vi "Main_21a.vi"() -> ()   [LabVIEW 2023]
uses:
  Cluster_Node.ctl
  ENUM Tile Marks.ctl
panel:
  out "Array":T1[][](array[typedef])
  out "Start Point":T2
  out "Answer":i32
  in  "Puzzle":string="...................................................................................................................................\n.....#..#..#.#..#..#..#................##.#.......#....................#......#.##...........#.....##...................#........#.\n.....#.#.............#.............#.....#.........#..................................#......#....#...##...#.#........#......###...\n.......#...#................#.......#....#.....#...#.......................#......#...#.##...#.....#.........#.......#.#...........\n.##.............#...................#...#......#........#.........................#...#........#....#....#.........#..........#....\n.....#..##....#..#...#......##......#.................................................#.#.....#......#......#.#.##.................\n..............#......#......#................#.................#.................#................#..#...#........##.............#.\n..........##..........##.......#.#.....#..........#...#.........#.....................#....#....................#..#.....##..#..##.\n.#.#..#..#.#....#....#.....#...#.#.................................................#......................#..##..#.........#...#...\n.....................#.........#.......###..#......................#...........####........##.......#.#.#......#.#....##.....#...#.\n.#.#...#....#.........##...#...........#..##.......#.......#.......#................#.....#...#...#.#.....#..............##......#.\n................#...#..#.........#.##............................................#......##.....##.......#...#........#..#..#.......\n..#..#..####...###.#..........#........#.......#.............#.....#....#............#..#........##......##.......#.....#....#.....\n.......#..........#.......................#.............##..........#..#..........#.....#.............##.........#..............#..\n..................#.............##...........................#.#......##.......................##.....#.#.....#................#...\n.......#...................##........#...............................#..............#..#..#.#..#..........#........#...........#...\n...#..........#..#...#.#.#............................#......................#.......#......##...#...............#...#..#..........\n...#.#..........#.#.....#........#.....#...#.......................#.....#..#...............#.....#.#......#....##...#....#..###...\n...#.##........#..##...#..........#..#..................................#..#.#.#.........#...........#....#.....#...#.#.........#..\n.....#.......#........#..............#.##.............#..#........#....#.....#.............#....#.#.#........##........#...#..#....\n....#......##....##........#..#....##.................#......................#.#.#................#....#..###..#...#...............\n....#....#.#........#.......#........#...................#.....#.........#....#............##.........#..............#...........#.\n............#..#.##..................#..........##.........................#..#....#................#................#..#....#.....\n.##.##........#..###.......#....#......................##..#......#.....#...#..#...............##.#.....##........#................\n.......#..#........#.........#...................#..#.....##...............#.#.#...#..........#............#.....##.........#......\n...###.......#...............#...................#..#...##.........#.............##..#..........................#..#...#.....#.....\n..#..............##.........#..#...............................#........#......#.#....#..........#................##.#...#.........\n...#......#..#....#.........#..#..........##............#....#.........#....#..#......#.........#..#...........#...................\n.#...###.....................#.............#.......#......###..#...........#.........................#..#.......#.#..#.....#.......\n.###........#......##...#...........................##......#.........#.........#........#........#.....##..........#....#.........\n.......#........#..#......#..............#..........##...#...#...........................#...........#...#..#......#...........#...\n.#....#........#......#..##..................#....................#.................................#......#.....#..#.......#......\n...#........#.....#..##...#.#.............#...#.#.#.....#......#........#...........#....#...............#..#.....#.......#........\n....#....#...#.#....#................#..#......#........#.#........#..#.#..#..#.....#..#..................##...................#...\n.......##........#...#..............###.#....#....#..#....##...#....##.#............#..#.#...#............#...................#.#..\n..#......#.........#..#.................#...#.......#....#...#..............##...#..........#.#...........................#....#...\n..#......#..#...........................#...........#....#.............#.#.........#...#.........................##............#...\n.....#................#.........#.#.........#...........#.#............#..................#....#.........................#..#..#...\n......#...#....##...................#.................#..#........#..#..#.....................#.............#.......#..#......#....\n.............##.................#.......#.........#..#....#...#.......#...................#.........#.......##.#...................\n......#....#.................#..#....#..##..#............#..............#.............#.....#..#..#................#..#...#......#.\n..................#.........#.....................#......#....##..##...##..........#......#......#..#.............#.....#....#.....\n.......#...#..#....#..........#.......#.#.#...##.....##.#....#.##..................##........#...##..................#.............\n.............#...#..................#......##.........#.......##......#...#....##.....#...#..#...................#...####..........\n.............................#.......#....#........#..........#...#.......#.#............#..###........#...........#.#.............\n..........#...................#..#...............#.#..................#.....#...#..............................................##..\n.........................................#...#.#....#.......#........#..#......#.........#...............#.........................\n......#...#.......................#.....#................#.........#..#......#....................####.#..#.....................##.\n.......#...................#.##....#......#..........#...............##...#...#...............#.......#.....#.................#....\n....#.#...##............#.......#..........#..................#..........#.........#........#.........##...#.......................\n...#......#.........#........#....#.....#.........#....##....#..................#.......#.#.........#.#..................##....#...\n.....#................#.#...........#.............#..#.......#..........#..#...#.#.....###......##.....#.#.#.#.................#...\n.....................#..##.##...#...............#..#....#....#....#..####...#..................................#.........##..#.....\n.......##...............#......#.....#..........#..#..#.#.............#.....#......#.#.......#..................#............#..##.\n...#............#...#.........##............#...#...#......#.......#.....#...##...##...#...#................................#......\n...#.#.............................................##..............##..................#...........#...#..........#...........##...\n...#.#....................#......#....#.....##..........#.........#......#.#.......##.#.#....#.#....#.....#....##..................\n.............#...#.#..#......#........#.#...##.#...............#....#.........................#....#.......#.....##...#.........#..\n..................##..#..###......................#.......#.##.....#....#..#.....#....#..............#.....#.#..#....#.............\n.............#......#.###..###........#.#.#......#.#....#..#.......#..#............#.........#.#..#...............#.............##.\n.............#...#.............#.#.#..##..####..#......#.##.#...........##...##.............#......#.............#..#............#.\n..........#........#......#.#........#..............#......#..#.#.....#.................#...#...............#.#..........##........\n..............#.............##.....#............................#..........#..........#..#.....................#..#..#.............\n..........#...#.#.......##....#.......#..##......#...#.....#............#................#....#.......................#............\n....................#.....#..........#.......#.#........#...##..............#.....#.......#..##...#..#####.#.#.........##....#.....\n.................................................................S.................................................................\n........#.........##....#........#...........................##........#..............#........#.....#.#..............#....#.......\n......#............#.............#............#.##...........#..#.....#....#.....#......#.#.#.......#.#.#...#......................\n............................#.........#........###........#...#....#.........#................#..#.............#....#..............\n............#......##..##.##...##.............#.........#............#.###.....#..................##..................#..#.........\n..............#......#................#...............#.....##..#..........#.....#..#..........#...........#.......................\n.........................#...........#..#......#.............#..#....#.......#..#.....#...#.............................#........#.\n...........##.....##.................#..........#.#.#..............#.....#.........#............#.................#................\n.........................#......#.....#...#.##...........#......#....#....#......#..#.#..#..###..##.##.....#...................#...\n.....#...........#.....#.......#..##......##.#.#.#..........#..#..............#...#.#.#.....#............#.#....#..............#.#.\n...#...........#.........#..#.#.#.........#........#..#........................#..........#.............#....##.#...............#..\n...............#.....................................#..............................##...###.................#..#..........#.....#.\n........#..........#..#......###............#........................#..........#............................................#.....\n...............................#....................#..................................##.............#............................\n.........#............#..#..........#........#..#...##....#....#..#......#.....#.#...#......................##..................#..\n......##.#..........##.#..................................#.........#......##..#...............#........#.....#............#.......\n.........#..................#...........#.#.......................#..........#.......##.......#.....#...##...#........#...#.#......\n...#...................#.....#...........##............#..#...#..................#.#..........#........................#...........\n..#.........#.........#.........##...#.....#...........#.....................#....#............#..#.......#.........#.....#........\n..........#....#..........#.........#..........#..###........#.#..........##.................#......#...#..............#...........\n..#....##..........................#..........#........#.#..##..#.....#.#....#..#.....................#............#.#...........#.\n.....................................#..#.#..#...........#...#.#.......#........#...#.........#...#..#...............#.............\n.........#.#....##.................#.#.....#....#..#..#................#...##.......#...........#.....#.................##.........\n..#.........................#......#..............#.............#.......#.............#........#................#...###.#........#.\n.#..#............#..............#..#...........#................#.........#....#................#..#.............#.....#...#.....#.\n.....#.......................#............#...............#..........###.....##...........#..#...#.##.........#.......#............\n.#..#..........#.............................#......#.......##..........#.........#....#...#.....#..........#....#.................\n.........#.......................#.##.....#.....#.#....#.......##.....#....#......#.......#.#.....................#.##..#..#....#..\n.#......#.....#.....#.....................##.........#....#...##..#..................##...#.#.#..#........#..#.........#.#....#.##.\n.#...............................#.#.#..#..##.....#........#...#.....#..#...#......#.#....#...##..................#................\n...........#......#...............#.....#.....#..##.........##........#.....#.........#...#..#............#.#.#...........#........\n..#............#..##..#..#..........#...#.......#.........#.......#.....#............................................#....#...#.#..\n....#...........#....................#............................#.#...#...............#.#..#.....................................\n.....##......#.##...#............................#........#...#...........#.........#......##...........#.#..#...............#.....\n......#..............##.#.###...........#.....#.#.##....#..#..........#...#..#..............................#.....#..............#.\n..##.....................##...............#...#......#........#..................#............................#.###..#...#....#..#.\n........#.#............#....................##.....#..........#...................#...#..#...........#........#.........#....##....\n.....#....#..#...............#............#.....#.......#...#........#............#..##.............#.......................#......\n..#.........#.............#...........................#.......#.#.................#..###.........................#.#.#.#.....#.....\n....#...#.................#................#........#..........#..........#.......#..........................#.#......#.......#....\n......#..##........#....#........................#.........#.........#................#......................#........#.....#....#.\n............#......#.........................................##......#.#..#.........#.............##..........#............#.......\n......#.#....#....#......#......##................#........#......#....#.....#....#.#..............#.......#.#...#......#......#...\n.....#............##.....#........#.#..#.........#.#................#...#.........#...........#.....#..#............#.....#..#.#...\n.......##..#........#..#..#.......................#............................................................#...#.#.....#.......\n....#...............#.......#............#.................#..............#..#...........#.......#............#................#...\n.......#.........##.......................#.......#....#......###...#....#..#................##...#.................#.#............\n...#.#.......#........#..#...........................#......#.....#.........##..........#..........##..............#....#........#.\n..#.#...........##..........#...#.........#..........#.#............##..................................#...........##.............\n.#..............#.........##.#.##..#...#....#.............#..............#............#..................#.#........#..............\n..#..#.....#....#.........#..#.#......#..#...#.............#..........#.................#...##.....#..........#...............#....\n......#.........#..#.#.....#................#......................#...##...........#..#................#.............#....##....#.\n...................#.....#.........##.....##...........................#....................#......#..................#..#.#.......\n..#............#...........##.#................................#............................#.........................#...#....#...\n.....#............#..............#......#..#....................#............................#....#....................#....#..#...\n..........#..#.#.#..............#.................................................................#...............##...........#...\n........##.................#..........#.....##....#.........#..#...#.##.....................#..#.........................#.......#.\n....##.........#.....#.....................#..#.##...........#..#.........................#..........#.....#........#....##......#.\n..............#.......#........#.......#..##...................#...#....................#...........#....#.........................\n...............#.............##......#.##.#............#...................#....#..............#...#..#.#.....#...............#....\n.....#..............#...#.......##..........#......#...#..................#..................#........#....#.........#.............\n.#.......#.#......#........................#..#......#......................#......##....##..#..........#...................#......\n..........#...........#..#..###........#.#......#.....................................#####.......##........#.....#.......#........\n..##................#............#..........#...##....#........................#....#........#....#.##......#.........##....#......\n.........#....#.....#....#.#...##..........#.........#.#.................##..............#..#......#.......#...#..............#.#..\n..................................................................................................................................."
  in  "Example":string="...........\n.....###.#.\n.###.##..#.\n..#.#...#..\n....#.#....\n.##..S####.\n.##..#...#.\n.......##..\n.##.#.####.\n.##..##.##.\n..........."
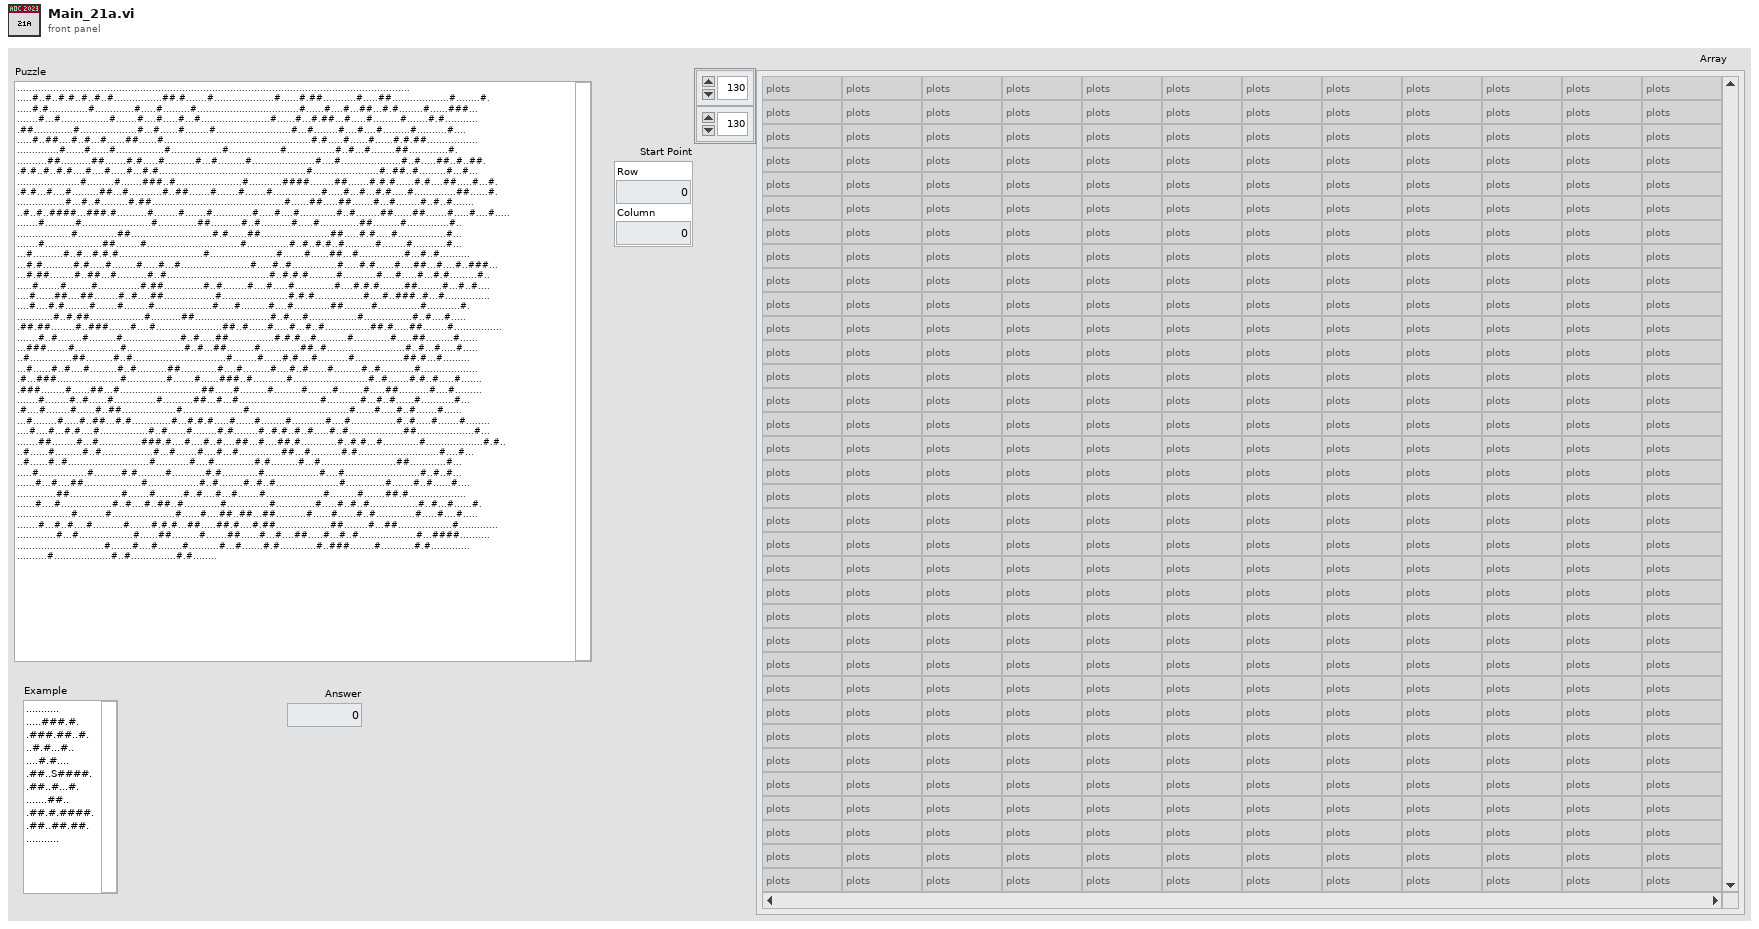
[diagram p1: front panel]
types:
  T1 = typedef "ENUM Tile Marks.ctl" = enum16{"plots", "rocks", "Start", "Marked Tiles"}
  T2 = typedef "Cluster_Node.ctl" = cluster{"Row":i32, "Column":i32}
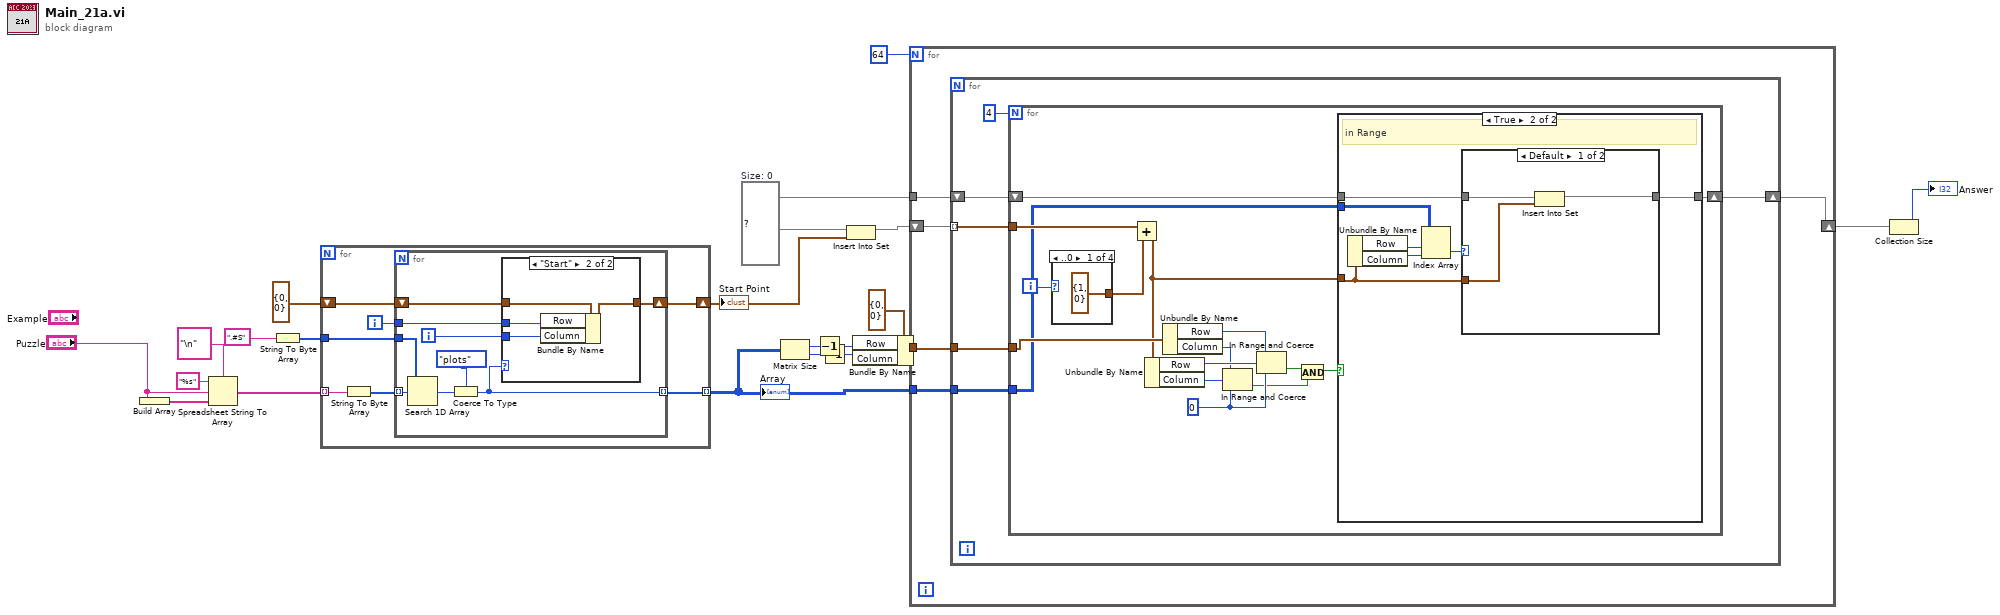
[diagram p0: block diagram]
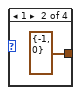
[diagram p4: hidden frame]
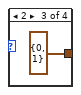
[diagram p5: hidden frame]
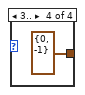
[diagram p6: hidden frame]
diagram:
  w4 = set{T2} {}  # Size: 0
  n1 = Build Array("Puzzle") -> (w21:string[])
  n2 = Spreadsheet String To Array(delimiter (Tab)="\n", format string="%s", spreadsheet string="Puzzle", array type (2D Dbl)=w21) -> (array=w18:string[])
  n3 = String To Byte Array(string=".#S" ("format string")) -> (unsigned byte array=w16:u8[])
  n4 = for {
    tunnel: w18 -> [w28] mode=indexing
    tunnel: w16 -> [w27]
    tunnel: [w25] -> w11 mode=indexing
    shift-right: [w22] -> w12
    shift-left: T2 {"Row"=0, "Column"=0} ("Point") -> [w24]
    i -> [w23]
    n5 = String To Byte Array(string=w28) -> (unsigned byte array=w26:u8[])
    n6 = for {
      tunnel: w27 -> [w37]
      tunnel: w26 -> [w36] mode=indexing
      tunnel: [w33] -> w25 mode=indexing
      shift-right: [w29] -> w22
      shift-left: w24 -> [w32]
      tunnel: w23 -> [w31]
      i -> [w30]
      n7 = Search 1D Array(1D array=w37, element=w36) -> (index of element=w35:i32)  [unwired: 1 in]
      n8 = Coerce To Type(0:w35, 1:ENUM_Tile_Marks."plots") -> (2:w33:T1)
      n9 = case shown="\"Start\"" w33 {
        tunnel: w32 -> [w38 w42]
        tunnel: w31 -> [_ w40]
        tunnel: w30 -> [_ w39]
        tunnel: [w38 w41] -> w29
        frame Default {
        }
        frame "Start" {
          n10 = Bundle By Name(cluster=w42, "Row"=w40, "Column"=w39) -> (w41:T2)
        }
      }
    }
  }
  "Start Point" <- w12
  "Array" <- w11
  n11 = Matrix Size(0:w11) -> (1:w9:i32, 2:w8:i32)
  n12 = Decrement(x=w9) -> (x-1=w6:i32)
  n13 = Decrement(x=w8) -> (x-1=w7:i32)
  n14 = Insert Into Set(10:w12, 11:w4) -> (3:w13:set{T2})  [unwired: 1 out]
  n15 = Bundle By Name(cluster=T2 {"Row"=0, "Column"=0} ("Start Point 2"), "Row"=w6, "Column"=w7) -> (w5:T2)
  n16 = for {
    N: 64 -> [_]
    tunnel: w11 -> [w45]
    shift-right: [w43] -> w3
    shift-left: w13 -> [w47]
    tunnel: w5 -> [w46]
    tunnel: w4 -> [w44]
    n17 = for {
      tunnel: w47 -> [w52] mode=indexing
      tunnel: w46 -> [w51]
      tunnel: w45 -> [w50]
      shift-right: [w48] -> w43
      shift-left: w44 -> [w49]
      n18 = for {
        N: 4 -> [_]
        tunnel: w52 -> [w68]
        tunnel: w51 -> [w63]
        tunnel: w50 -> [w57]
        shift-right: [w54] -> w48
        shift-left: w49 -> [w55]
        i -> [w69]
        w64 = 0
        n19 = case shown="..0" w69 {
          tunnel: [T2 {"Row"=1, "Column"=0} ("Start Point 2") T2 {"Row"=-1, "Column"=0} ("Start Point 2") T2 {"Row"=0, "Column"=1} ("Start Point 2") T2 {"Row"=0, "Column"=-1} ("Start Point 2")] -> w67
          frame ..0 {
          }
          frame 1 {
          }
          frame 2 {
          }
          frame 3.. {
          }
        }
        n20 = Add(x=w68, y=w67) -> (x+y=w56:T2)
        n21 = Unbundle By Name(w56) -> ("Row"=w66:i32, "Column"=w65:i32)
        n22 = Unbundle By Name(w63) -> ("Row"=w61:i32, "Column"=w62:i32)
        n23 = In Range and Coerce(upper limit=w62, x=w65, lower limit=w64) -> (In Range?=w59:bool)  [unwired: 1 out]
        n24 = In Range and Coerce(upper limit=w61, x=w66, lower limit=w64) -> (In Range?=w60:bool)  [unwired: 1 out]
        n25 = And(x=w60, y=w59) -> (x .and. y?=w58:bool)
        n26 = case shown="True" w58 {
          tunnel: w57 -> [_ w77]
          tunnel: w56 -> [_ w71]
          tunnel: w55 -> [w70 w73]
          tunnel: [w70 w72] -> w54
          frame False {
          }
          frame True {
            # "in Range"
            n27 = Unbundle By Name(w71) -> ("Row"=w76:i32, "Column"=w75:i32)
            n28 = Index Array(array=w77, index (row)=w76, index (col)=w75) -> (element=w74:T1)
            n29 = case shown="Default" w74 {
              tunnel: w73 -> [w80 w81]
              tunnel: [w79 w81] -> w72
              tunnel: w71 -> [w78 _]
              frame Default {
                n30 = Insert Into Set(10:w78, 11:w80) -> (3:w79:set{T2})  [unwired: 1 out]
              }
              frame "rocks" {
              }
            }
          }
        }
      }
    }
  }
  n31 = Collection Size(1:w3) -> (0:→"Answer":i32)
